vi "PH_Calorimeter_USB.set modified data.vi"(0 "i ref in":refnum<vi>, 2 "i attribute":T1={"GUI Refs"={"Delete"=refnum, "Start"=refnum, "Energy"=refnum, "Calorimeter"=refnum, "Trigger"=refnum, "Calo Calibration"=refnum, "Time Base"=refnum, "Device"=refnum, "Graph Raw Data"=refnum, "Graph Result"=refnum}, "DAQ Instance"="N/A", "Data"=[], "Controller Instance"="N/A", "Energy [J]"=0.0, "Calorimeter"={"Channel"="Dev1/ai1", "Min Value [V]"=-1.0, "Max Value  [V]"=1.0}, "Trigger"={"Channel"="", "Min Value [V]"=-10.0, "Max Value  [V]"=10.0, "Level [V]"=1.0, "Wait Time [s]"=60.0, "Length [Samples]"=10}, "Time Base"={"Samples per Channel"=28000, "Rate [Hz]"=-1}, "Calo Calibration"={"T 1/e [s]"=220.0, "Sensitivity  [Vs/J]"=-10.0}, "Serial Number"="N/A"} {"Calo Calibration"."Sensitivity  [Vs/J]" format="%.4f"; "Trigger"."Level [V]" format="%0.2f"; "Trigger"."Max Value  [V]" format="%0.2f"; "Trigger"."Min Value [V]" format="%0.2f"; "Calorimeter"."Max Value  [V]" format="%0.2f"; "Calorimeter"."Min Value [V]" format="%0.2f"}, 5 "error in (no error)":errorcluster) -> (14 "i ref out":refnum<vi>, 19 "error out":errorcluster)   [LabVIEW 2014, in "PH_Calorimeter_USB.lvlib"]
doc: "Writes the data into the attribute of an object. Then, the attribute dara are unlocked using the \"release\" method. Prior to calling THIS method, the attribute data must have been locked using the methods \"lock\" or \"get data to modify\".\n\n\nLicense Agreement for this software:\n\nCopyright (C)\nGesellschaft für Schwerionenforschung, GSI\nPlanckstr. 1\n64291 Darmstadt\nGermany\n\nContact: D.Beck@gsi.de \n\nThis program is free software; you can redistribute it and/or modify it under the terms of the GNU General Public License as published by the Free Software Foundation; either version 2 of the license, or (at your option) any later version.\n\nThis program is distributed in the hope that it will be useful, but WITHOUT ANY WARRANTY; without even the implied warranty of MERCHANTABILITY or FITNESS FOR A PARTICULAR PURPOSE. See the GNU General License for more details (http://www.gnu.org).\n\nGesellschaft für Schwerionenforschung, GSI\nPlanckstr. 1, 64291 Darmstadt, Germany\nFor all questions and ideas contact: M.Richter@gsi.de, H.Brand@gsi.de or D.Beck@gsi.de.\nLast update: 17-JUN-2004"
uses:
  PH_Calorimeter_USB.lvlib
  PH_Calorimeter_USB.i attribute.ctl
  PH_Calorimeter_USB.Calorimeter Settings.ctl
  PH_Calorimeter_USB.Trigger Settings.ctl
  PH_Calorimeter_USB.Time Base Settings.ctl
  PH_Calorimeter_USB.Calorimeter Calibration Settings.ctl
  CSCore/CSObj/CSObj.lvlib
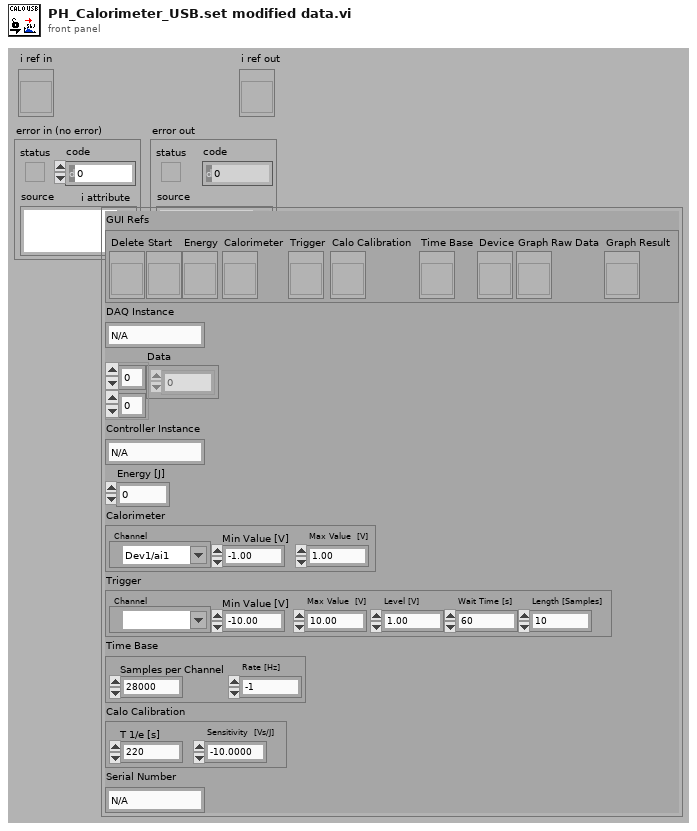
[diagram p1: front panel]
types:
  T1 = typedef "PH_Calorimeter_USB.lvlib/PH_Calorimeter_USB.i attribute.ctl" = cluster{"GUI Refs":cluster{"Delete":refnum<vi>, "Start":refnum<vi>, "Energy":refnum<vi>, "Calorimeter":refnum<vi>, "Trigger":refnum<vi>, "Calo Calibration":refnum<vi>, "Time Base":refnum<vi>, "Device":refnum<vi>, "Graph Raw Data":refnum<vi>, "Graph Result":refnum<vi>}, "DAQ Instance":string, "Data":dbl[][], "Controller Instance":string, "Energy [J]":dbl, "Calorimeter":T2, "Trigger":T3, "Time Base":T4, "Calo Calibration":T5, "Serial Number":string}
  T2 = typedef "PH_Calorimeter_USB.lvlib/PH_Calorimeter_USB.Calorimeter Settings.ctl" = cluster{"Channel":tag, "Min Value [V]":dbl, "Max Value  [V]":dbl}
  T3 = typedef "PH_Calorimeter_USB.lvlib/PH_Calorimeter_USB.Trigger Settings.ctl" = cluster{"Channel":tag, "Min Value [V]":dbl, "Max Value  [V]":dbl, "Level [V]":dbl, "Wait Time [s]":dbl, "Length [Samples]":i32}
  T4 = typedef "PH_Calorimeter_USB.lvlib/PH_Calorimeter_USB.Time Base Settings.ctl" = cluster{"Samples per Channel":i32, "Rate [Hz]":i32}
  T5 = typedef "PH_Calorimeter_USB.lvlib/PH_Calorimeter_USB.Calorimeter Calibration Settings.ctl" = cluster{"T 1/e [s]":dbl, "Sensitivity  [Vs/J]":dbl}
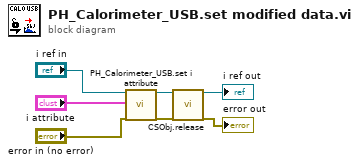
[diagram p0: block diagram]
diagram:
  n1 = call "PH_Calorimeter_USB.set i attribute.vi"("i ref in"="i ref in", "i attribute"="i attribute", "error in (no error)"="error in (no error)") -> ("i ref out"=w4:refnum<vi>, "error out"=w3:errorcluster)  [unwired: 15 in]
  n2 = call "CSObj.release.vi"("i ref in"=w4, "error in (no error)"=w3) -> ("i ref out"=→"i ref out":refnum<vi>, "error out"=→"error out":errorcluster)  [unwired: 16 in]
